vi "AT Open A.vi"(8 "error in (no error)":errorcluster, 10 "CameraIndex":i32) -> (0 "error out":errorcluster, 2 "Handle":i32, 3 "Status":i32)   [LabVIEW 2019]
doc: "Open\n\nOutput:\n I32 Status\n\nInput:\n void\n\nThis function is used to open up a handle to a particular camera. The DeviceIndex parameter indicates the\nindex of the camera that you wish to open and the handle to the camera is returned in the Handle parameter. This Handle parameter must be passed as the first parameter to all other functions to access the features or to acquire data from the camera."
uses:
  atcoreA.dll
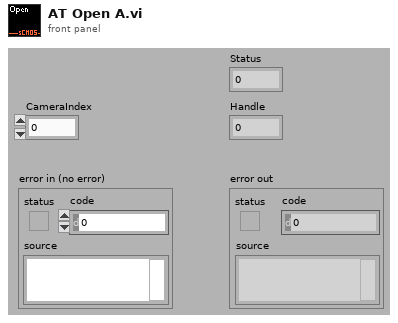
[diagram p1: front panel]
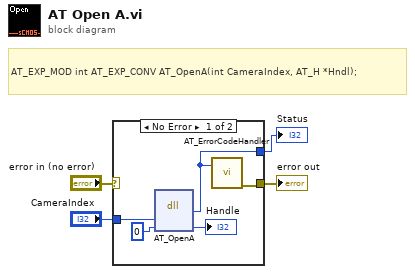
[diagram p0: block diagram]
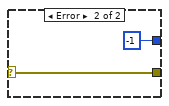
[diagram p2: hidden frame]
diagram:
  # "AT_EXP_MOD int AT_EXP_CONV AT_OpenA(int CameraIndex, AT_H *Hndl);"
  n1 = case shown="No Error" "error in (no error)" {
    selector: "error in (no error)" -> [_ w11]
    tunnel: [w5 -1 ("return type")] -> w4
    tunnel: "CameraIndex" -> [w9 _]
    tunnel: [w6 w11] -> w1
    frame No Error {
      n2 = dll-call lib="atcoreA.dll" fn="AT_OpenA"("CameraIndex"=w9, "Handle"=0 ("Hndl")) -> ("Status"=w5:i32, "Handle"=→"Handle":i32)  [unwired: 4 in, 2 out]
      n3 = call <userlib>:"AT_ErrorCodeHandler.vi"("Error"=w5) -> ("error out"=w6:errorcluster)  [unwired: 6 in]
    }
    frame Error {
    }
  }
  "Status" <- w4
  "error out" <- w1
